vi "PreChecks.vi"(8 "type":T1(ring), 9 "Y":dbl, 11 "X":dbl) -> (1 "message":string, 3 "Error":bool)   [LabVIEW 2014]
uses:
  <userlib>/Nanonis Prog Interface V5/Scan/Piezos/Piezo Calibration Range Get.vi
  <userlib>/Nanonis Prog Interface V5/Nanonis Prog Interface.lvlib
panel:
  in  "lower limit dip":dbl=-3e-08 format="%#_13p"
  in  "upper limit dip":dbl=3e-08 format="%#_13p"
  in  "upper limit bias":dbl=8.2 format="%#_13p"
  in  "lower limit bias":dbl=0.019 format="%#_13p"
  in  "upper limit time":dbl=5.0 format="%#_13p"
  in  "lower limit time":dbl=0.02 format="%#_13p"
  in  "pixel lower limit":dbl=8.0
  in  "pixel upper limit":dbl=1024.0
  in  "min image size":dbl=1e-09 format="%#_6p"
  in  "max image size":dbl=2e-07 format="%#_6p"
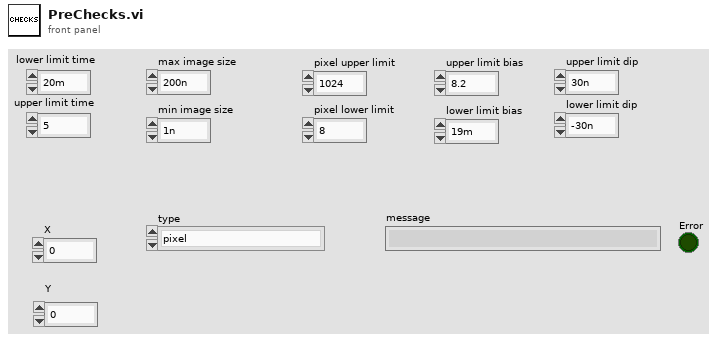
[diagram p1: front panel]
types:
  T1 = enum16{"pixel", "position", "size", "dip", "bias", "timing"}
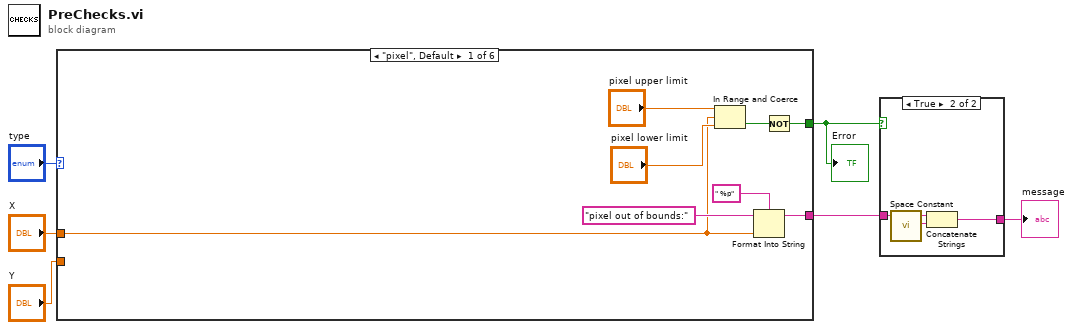
[diagram p0: block diagram]
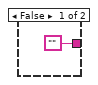
[diagram p2: hidden frame]
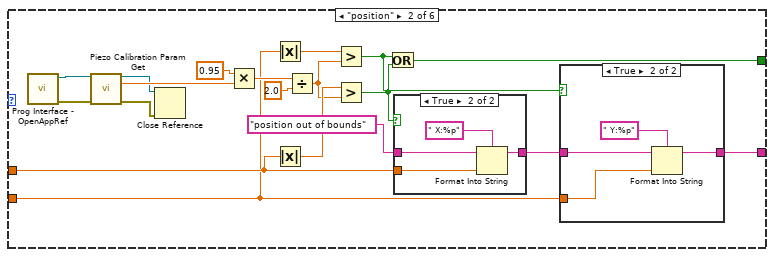
[diagram p3: hidden frame]
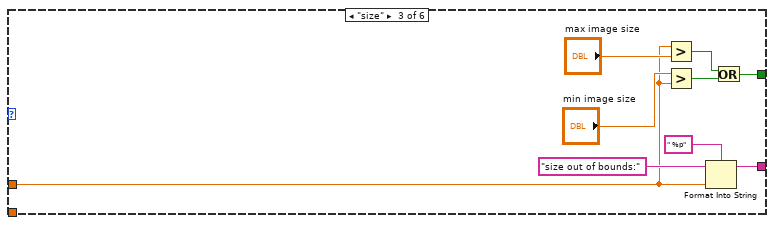
[diagram p6: hidden frame]
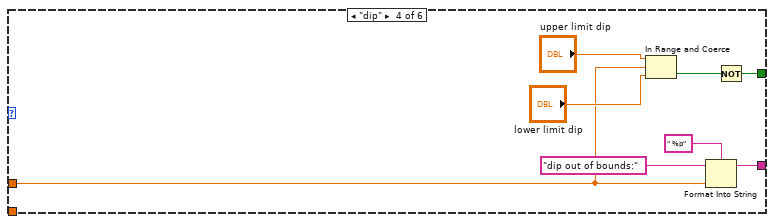
[diagram p7: hidden frame]
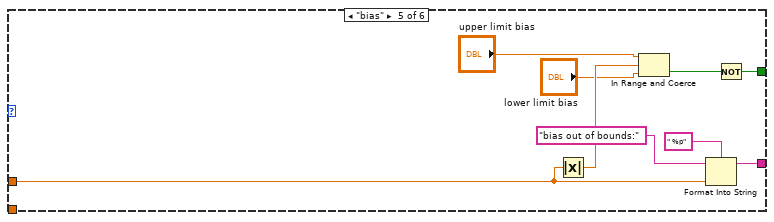
[diagram p8: hidden frame]
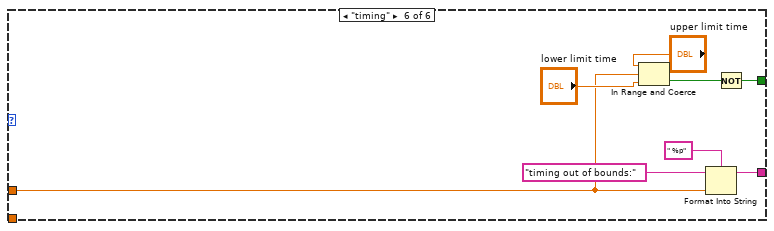
[diagram p9: hidden frame]
diagram:
  n1 = case shown="\"pixel\", Default" "type" {
    tunnel: "X" -> [w7 w21 w45 w53 w64 w70]
    tunnel: "Y" -> [_ w20 _ _ _ _]
    tunnel: [w11 w27 w50 w55 w68 w71] -> w3
    tunnel: [w8 w19 w44 w54 w65 w73] -> w2
    frame "pixel", Default {
      n2 = In Range and Coerce(upper limit="pixel upper limit", x=w7, lower limit="pixel lower limit") -> (In Range?=w12:bool)  [unwired: 1 out]
      n3 = Format Into String(format string=" %p", initial string="pixel out of bounds:" ("message"), w7) -> (resulting string=w8:string)  [unwired: 1 in, 1 out]
      n4 = Not(x=w12) -> (.not. x?=w11:bool)
    }
    frame "position" {
      n5 = call <userlib>:"Prog Interface - OpenAppRef.vi"() -> ("Error out"=w15:errorcluster, "Application reference"=w16:refnum<vi>)  [unwired: 6 in]
      n6 = call-poly <userlib>:"Piezo Calibration Param Get.vi"("Application ref in"=w16, "error in (no error)"=w15) -> ("Application ref out"=w18:refnum<vi>, "Range X (m)"=w26:sgl, "error out"=w17:errorcluster)  [unwired: 9 in, 2 out]
      n7 = Close Reference(reference=w18, error in (no error)=w17) -> ()  [unwired: 1 out]
      n8 = Multiply(x=0.95, y=w26) -> (x*y=w33:dbl)
      n9 = Absolute Value(x=w20) -> (abs(x)=w30:dbl)
      n10 = Absolute Value(x=w21) -> (abs(x)=w29:dbl)
      n11 = Divide(x=w33, y=2.0) -> (x/y=w28:dbl)
      n12 = Greater?(x=w30, y=w28) -> (0:w22:bool)
      n13 = Greater?(x=w29, y=w28) -> (0:w23:bool)
      n14 = Or(x=w22, y=w23) -> (x .or. y?=w27:bool)
      n15 = case shown="True" w23 {
        tunnel: "position out of bounds" ("message") -> [w39 w42]
        tunnel: [w39 w41] -> w24
        tunnel: w21 -> [_ w40]
        frame False {
        }
        frame True {
          n16 = Format Into String(format string=" X:%p", initial string=w42, w40) -> (resulting string=w41:string)  [unwired: 1 in, 1 out]
        }
      }
      n17 = case shown="True" w22 {
        tunnel: w24 -> [w34 w38]
        tunnel: w20 -> [_ w36]
        tunnel: [w34 w35] -> w19
        frame False {
        }
        frame True {
          n18 = Format Into String(format string=" Y:%p", initial string=w38, w36) -> (resulting string=w35:string)  [unwired: 1 in, 1 out]
        }
      }
    }
    frame "size" {
      n19 = Greater?(x=w45, y="max image size") -> (0:w52:bool)
      n20 = Greater?(x="min image size", y=w45) -> (0:w51:bool)
      n21 = Format Into String(format string=" %p", initial string="size out of bounds:" ("message"), w45) -> (resulting string=w44:string)  [unwired: 1 in, 1 out]
      n22 = Or(x=w52, y=w51) -> (x .or. y?=w50:bool)
    }
    frame "dip" {
      n23 = In Range and Coerce(upper limit="upper limit dip", x=w53, lower limit="lower limit dip") -> (In Range?=w56:bool)  [unwired: 1 out]
      n24 = Format Into String(format string=" %p", initial string="dip out of bounds:" ("message"), w53) -> (resulting string=w54:string)  [unwired: 1 in, 1 out]
      n25 = Not(x=w56) -> (.not. x?=w55:bool)
    }
    frame "bias" {
      n26 = Absolute Value(x=w64) -> (abs(x)=w63:dbl)
      n27 = In Range and Coerce(upper limit="upper limit bias", x=w63, lower limit="lower limit bias") -> (In Range?=w69:bool)  [unwired: 1 out]
      n28 = Format Into String(format string=" %p", initial string="bias out of bounds:" ("message"), w64) -> (resulting string=w65:string)  [unwired: 1 in, 1 out]
      n29 = Not(x=w69) -> (.not. x?=w68:bool)
    }
    frame "timing" {
      n30 = In Range and Coerce(upper limit="upper limit time", x=w70, lower limit="lower limit time") -> (In Range?=w72:bool)  [unwired: 1 out]
      n31 = Format Into String(format string=" %p", initial string="timing out of bounds:" ("message"), w70) -> (resulting string=w73:string)  [unwired: 1 in, 1 out]
      n32 = Not(x=w72) -> (.not. x?=w71:bool)
    }
  }
  "Error" <- w3
  n33 = case shown="True" w3 {
    tunnel: ["" w80] -> w1
    tunnel: w2 -> [_ w81]
    frame False {
    }
    frame True {
      n34 = call <vilib>:"Space Constant.vi"() -> ("String"=w79:string)
      n35 = Concatenate Strings(w81, w79) -> (w80:string)
    }
  }
  "message" <- w1
